vi "Read_offsets_from_DB.vi"(8 "Assembly date":timestamp=timestamp(3857862657.9114094 s since 1904-01-01) format="%<%Y-%m-%d>T", 9 "PUT position":string, 10 "Assembly Tray ID":string, 11 "Module?":bool) -> (1 "ang_offset_deg":dbl[](array[numeric]), 2 "y_offset_mm":dbl[](array[numeric]), 3 "x_offset_mm":dbl[](array[numeric]))   [LabVIEW 2021, in "Pick and Place.lvclass"]
uses:
  Pick and Place.lvclass
  <vilib>/Utility/file.llb/Read Delimited Spreadsheet (string).vi
panel:
  out "last mod":timestamp
  out "error out (filesystem)":errorcluster
  in  "error in (filesystem)":errorcluster
  out "ass_tray_ids":string[](array[string])
  out "put_positions":string[](array[string])
  in  "No of modules requested":dbl
  out "No of returned entries":dbl
  out "Date text":string
  out "error out py":errorcluster
  in  "error in (no error) py":errorcluster
  out "DB offsets out":string[][](array[string])
  # "If no of modules requested is 0, it will return all modules"
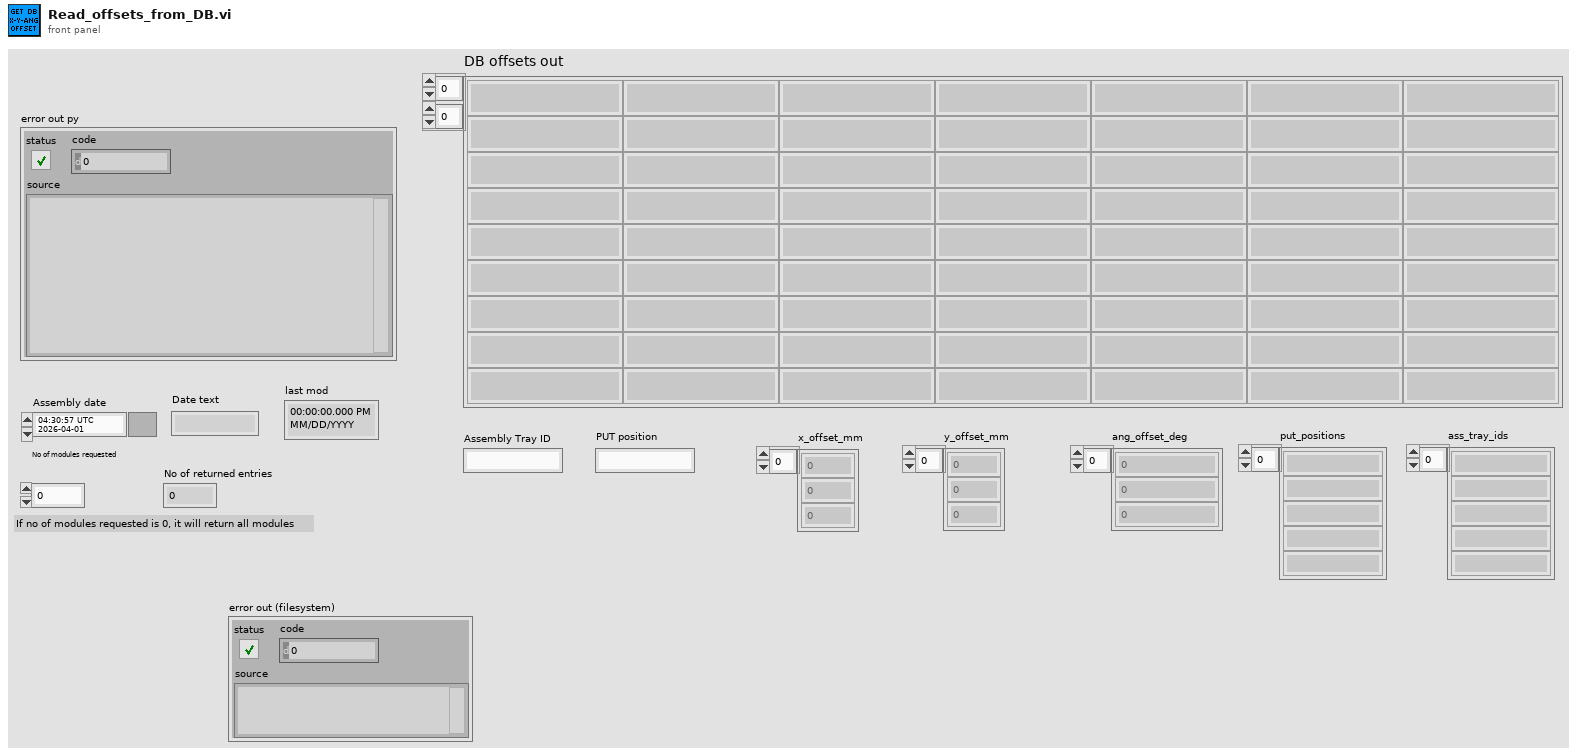
[diagram p1: front panel]
types:
  T1 = typedef "File Paths.ctl" = cluster{"Glue Pattern Folder":path, "Carrier Tray Folder":path, "Pick Up Tool Fixture Folder":path, "Components Folder":path, "Bellows Tool Offset.txt":path, "Pick Up Tool Offset.txt":path, "Dispense Tip Offset.txt":path, "Log Files":path, "Gantry Assembly Map.txt":path, "Syringe and offset map.txt":path, "Controllers Folder":path, "Local dbase config":path}
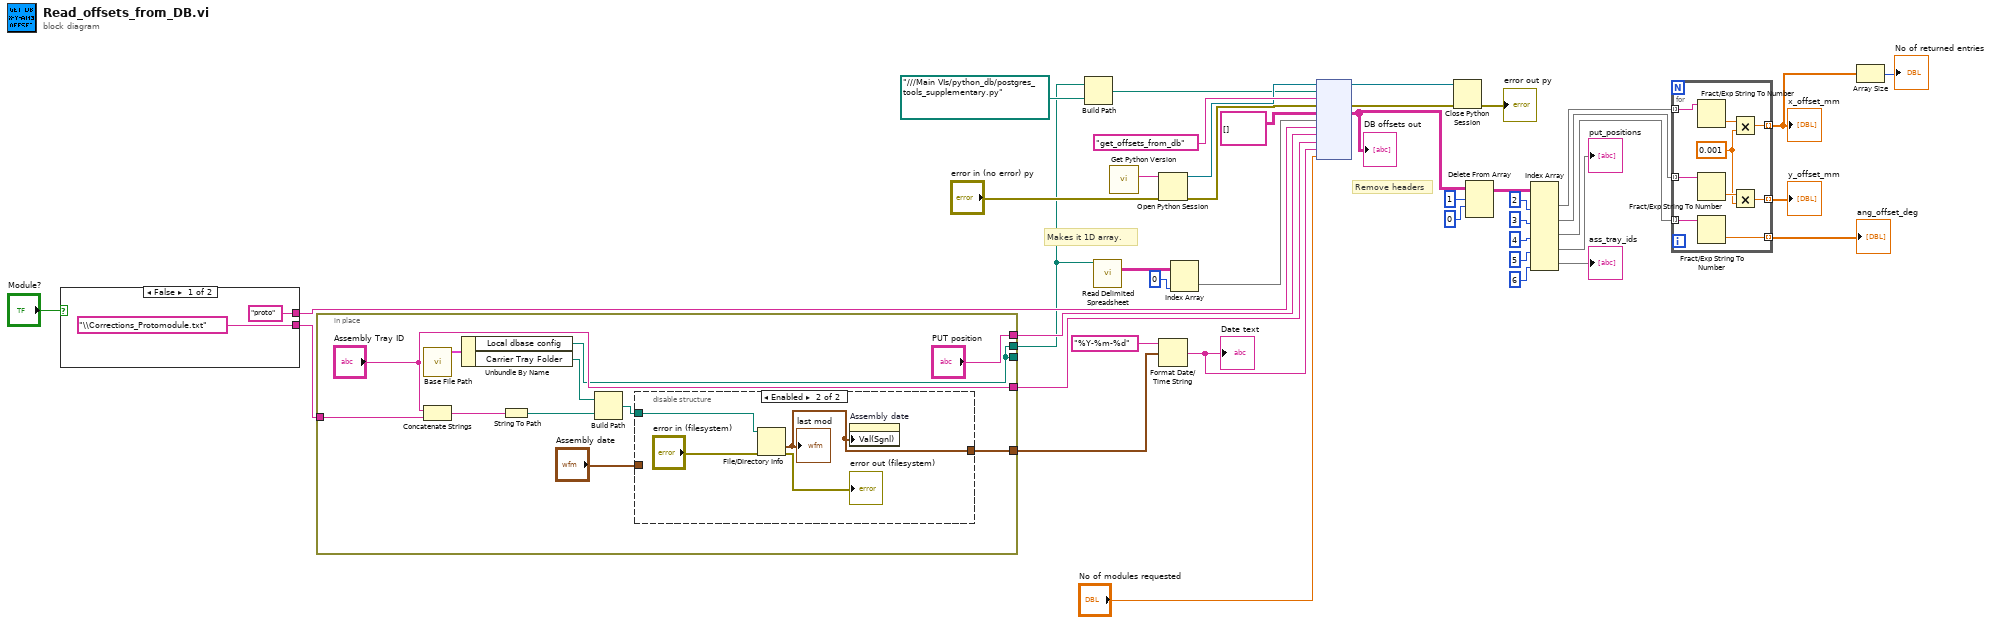
[diagram p0: block diagram]
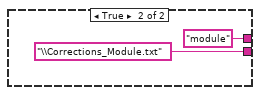
[diagram p3: hidden frame]
diagram:
  # "Remove headers"
  # "Makes it 1D array."
  n1 = case shown="False" "Module?" {
    tunnel: ["proto" "module"] -> w30
    tunnel: ["\\Corrections_Protomodule.txt" ("string") "\\Corrections_Module.txt" ("string")] -> w14
    frame False {
    }
    frame True {
    }
  }
  n2 = in-place {
    in-place-border: [w50] -> w2
    in-place-border: w14 -> [w54]
    in-place-border: ["Assembly Tray ID"] -> w7
    in-place-border: ["PUT position"] -> w6
    in-place-border: [w50] -> _
    in-place-border: [w47] -> w4
    n3 = call "Base File Path.vi"() -> ("Paths Out"=w57:T1)  [unwired: 11 in]
    n4 = Concatenate Strings("Assembly Tray ID", w54) -> (w55:string)
    n5 = Unbundle By Name(w57) -> ("Local dbase config"=w50:path, "Carrier Tray Folder"=w56:path)
    n6 = String To Path(string=w55) -> (path=w53:path)
    n7 = Build Path(base path=w56, name or relative path=w53) -> (appended path=w49:path)
    n8 = disable-structure shown="Enabled" {
      disable-tunnel: [w58 w59] -> w47
      disable-tunnel: w49 -> [_ w60]
      disable-tunnel: "Assembly date" -> [w58 _]
      frame Disabled {
      }
      frame Enabled {
        n9 = File/Directory Info(path=w60, error in="error in (filesystem)") -> (last mod=w59:timestamp, error out=→"error out (filesystem)":errorcluster)  [unwired: 5 out]
        "last mod" <- w59
        n10 = property on="Assembly date" class="AbsTime (strict)"("Val(Sgnl)"=w59) -> ()  [unwired: 2 in, 2 out]
      }
    }
  }
  n11 = Build Path(base path=w2, name or relative path=path "../../../Main VIs/python_db/postgres_tools_supplementary.py" ("module path")) -> (appended path=w1:path)
  n12 = call-poly <vilib>:"Read Delimited Spreadsheet.vi"("file path (dialog if empty)"=w2) -> ("all rows"=w39:string[][])  [unwired: 9 in, 5 out]
  n13 = call "Get Python Version.vi"() -> ("Python Version"=w38:string)  [unwired: 10 in, 1 out]
  n14 = Open Python Session(python version=w38, 3:"error in (no error) py") -> (session out=w35:refnum<k35>, error out=w36:errorcluster)  [unwired: 1 in]
  n15 = Format Date/Time String(time format string (%c)="%Y-%m-%d", seconds (now)=w4) -> (date/time string=w8:string)  [unwired: 1 in]
  "Date text" <- w8
  n16 = Index Array(array=w39, index (col)=0 ("disabled index (col)")) -> (element=w33:string[])  [unwired: 1 in]
  n17 = node(w35, w1, "get_offsets_from_db" ("function name"), w36, string[][] [], w33, w30, w6, w7, w8, "No of modules requested") -> (w32:refnum<k35>, w31:errorcluster, w26:string[][])  [unwired: 6 in, 2 out]
  "DB offsets out" <- w26
  n18 = Close Python Session(session in=w32, error in=w31) -> (11:→"error out py":errorcluster)
  n19 = Delete From Array(array=w26, length=1, index (row)=0) -> (array with subset deleted=w25:string[][])  [unwired: 1 in, 1 out]
  n20 = Index Array(array=w25, index (col) #1=2 ("index (row)"), index (col) #2=3 ("index (col)"), index (col) #3=4 ("index (col)"), index (col) #4=5 ("index (col)"), index (col) #5=6 ("index (col)")) -> (element #1=w24:string[], element #2=w21:string[], element #3=w18:string[], element #4=→"put_positions":string[], element #5=→"ass_tray_ids":string[])  [unwired: 5 in]
  n21 = for {
    tunnel: w24 -> [w71] mode=indexing
    tunnel: [w66] -> w16 mode=indexing
    tunnel: w21 -> [w70] mode=indexing
    tunnel: [w64] -> w20 mode=indexing
    tunnel: w18 -> [w69] mode=indexing
    tunnel: [w68] -> w17 mode=indexing
    w63 = 0.001 ("y")
    n22 = Fract/Exp String To Number(string=w71) -> (number=w67:dbl)  [unwired: 3 in, 1 out]
    n23 = Fract/Exp String To Number(string=w70) -> (number=w65:dbl)  [unwired: 3 in, 1 out]
    n24 = Fract/Exp String To Number(string=w69) -> (number=w68:dbl)  [unwired: 3 in, 1 out]
    n25 = Multiply(x=w67, y=w63) -> (x*y=w66:dbl)
    n26 = Multiply(x=w65, y=w63) -> (x*y=w64:dbl)
  }
  "x_offset_mm" <- w16
  "y_offset_mm" <- w20
  "ang_offset_deg" <- w17
  n27 = Array Size(array=w16) -> (size(s)=→"No of returned entries":i32)
